vi "Read Timeout (ms).vi"(8 "error in (no error)":errorcluster, 11 "FPGA Serial Session in":refnum<class "FPGA Serial Session.lvclass">) -> (0 "error out":errorcluster, 2 "Timeout (ms)":i32=100, 3 "FPGA Serial Session out":refnum<class "FPGA Serial Session.lvclass">)   [LabVIEW 2015, in "FPGA Serial Session.lvclass"]
uses:
  FPGA Serial Session.lvclass
  FPGA Serial Session.lvclass/FPGA Serial Session.ctl
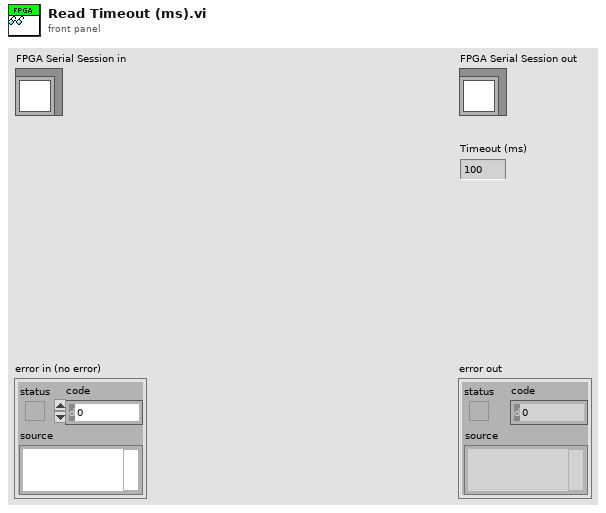
[diagram p1: front panel]
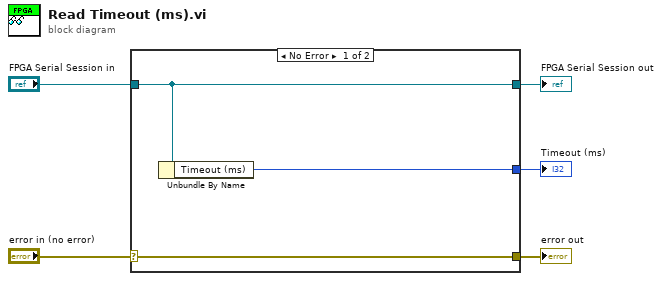
[diagram p0: block diagram]
diagram:
  n1 = case shown="No Error" "error in (no error)" {
    selector: "error in (no error)" -> [w8 w9]
    tunnel: [w8 w9] -> w4
    tunnel: [w7 w10] -> w2
    tunnel: "FPGA Serial Session in" -> [w7 w10]
    tunnel: [w6 _] -> w1
    frame No Error {
      n2 = Unbundle By Name(w7) -> ("Timeout (ms)"=w6:i32)
    }
    frame Error {
    }
  }
  "error out" <- w4
  "FPGA Serial Session out" <- w2
  "Timeout (ms)" <- w1
